vi "BFM.vi"(0 "in 0":T2, 1 "in 1":T2, 2 "in 2":T2, 3 "in 3":T2, 4 "in 4":T2, 5 "in 5":T2, 6 "in 6":T2, 7 "in 7":T2, 8 "in 8":T2, 9 "in 9":T2, 10 "in 10":T2, 11 "in 11":T2, 12 "in 12":T2, 13 "in 13":T2, 14 "in 14":T2, 15 "in 15":T2, 16 "in 16":T2, 17 "in 17":T2, 18 "in 18":T2, 19 "in 19":T2, 20 "in 20":T2, 21 "in 21":T2, 22 "in 22":T2, 23 "in 23":T2, 24 "in 24":T2, 25 "Func":T3) -> (27 "out":T1)   [LabVIEW 2013]
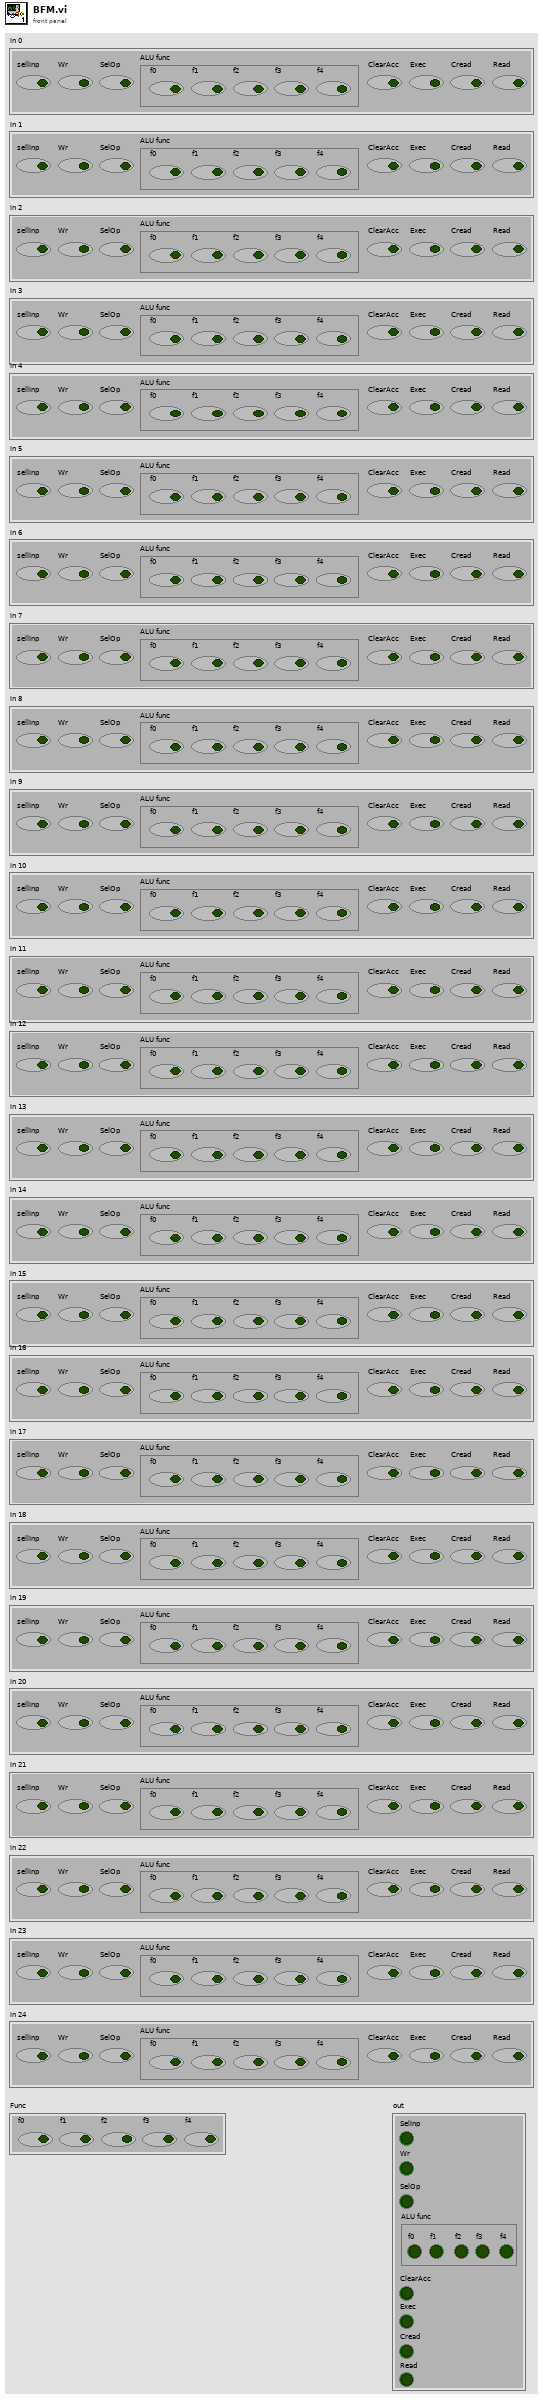
[diagram p1: front panel]
types:
  T1 = cluster{"SelInp":bool, "Wr":bool, "SelOp":bool, "ALU func":cluster{"f0":bool, "f1":bool, "f2":bool, "f3":bool, "f4":bool}, "ClearAcc":bool, "Exec":bool, "Cread":bool, "Read":bool}
  T2 = cluster{"sellInp":bool, "Wr":bool, "SelOp":bool, "ALU func":cluster{"f0":bool, "f1":bool, "f2":bool, "f3":bool, "f4":bool}, "ClearAcc":bool, "Exec":bool, "Cread":bool, "Read":bool}
  T3 = cluster{"f0":bool, "f1":bool, "f2":bool, "f3":bool, "f4":bool}
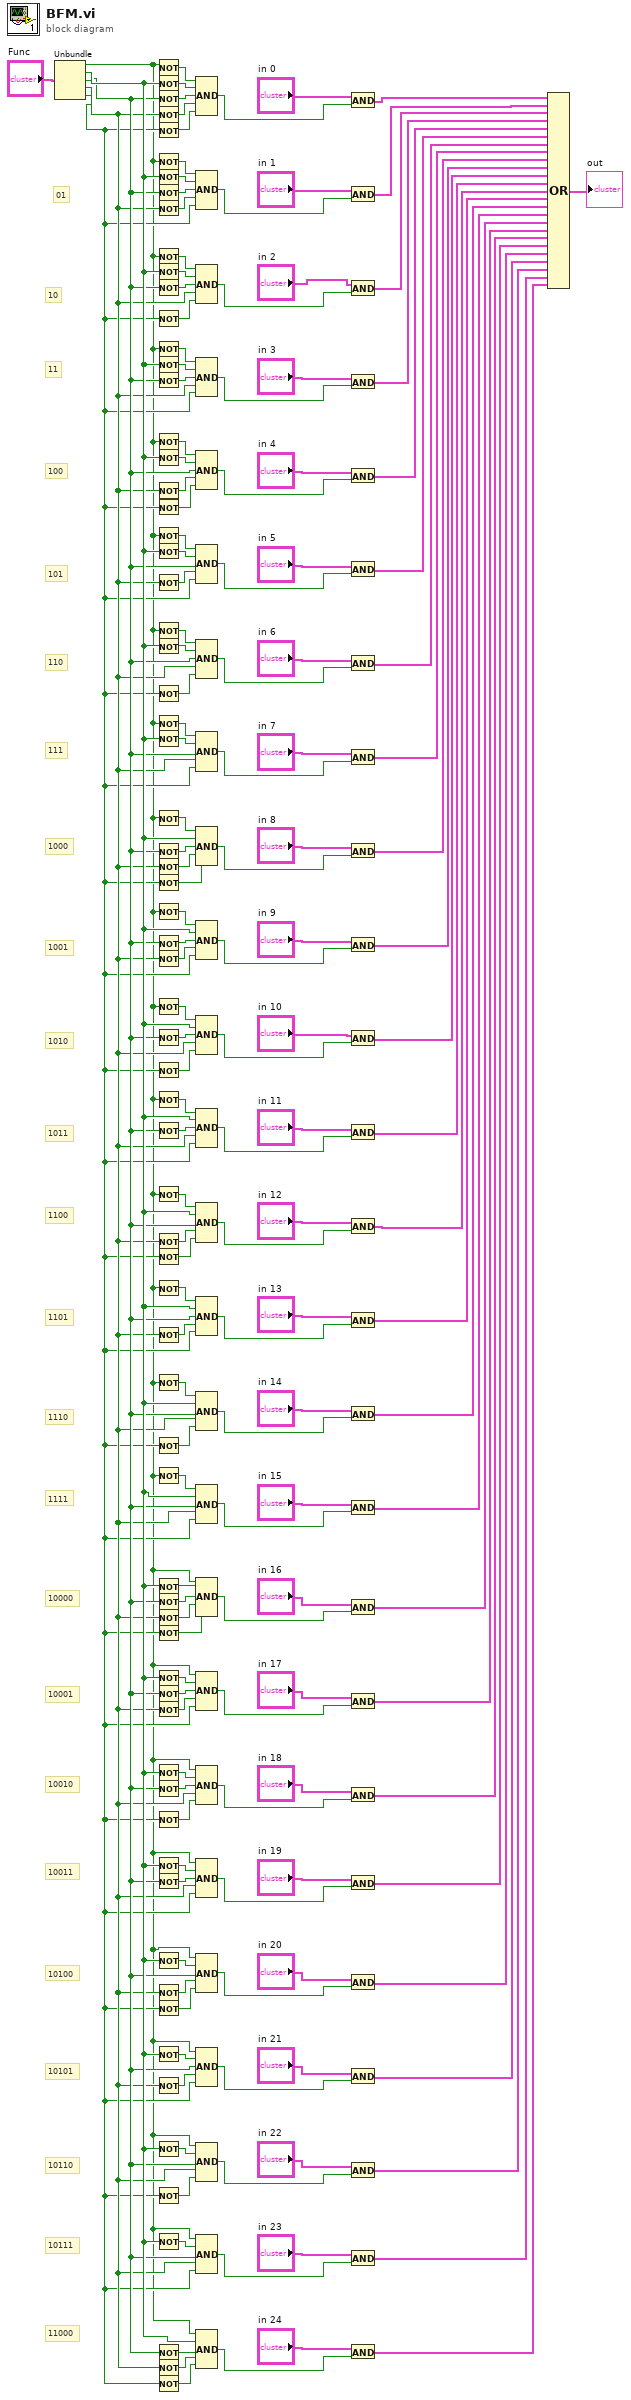
[diagram p0: block diagram]
diagram:
  # "01"
  # "11000"
  # "10111"
  # "10110"
  # "10101"
  # "10100"
  # "10011"
  # "10010"
  # "10001"
  # "10000"
  # "1111"
  # "1110"
  # "1101"
  # "1100"
  # "1011"
  # "1010"
  # "1001"
  # "1000"
  # "111"
  # "110"
  # "101"
  # "100"
  # "11"
  # "10"
  n1 = Unbundle("Func") -> ("f0"=w1:bool, "f1"=w8:bool, "f2"=w4:bool, "f3"=w3:bool, "f4"=w2:bool)
  n2 = Not(x=w1) -> (.not. x?=w94:bool)
  n3 = Not(x=w8) -> (.not. x?=w93:bool)
  n4 = Not(x=w4) -> (.not. x?=w90:bool)
  n5 = Not(x=w3) -> (.not. x?=w91:bool)
  n6 = Not(x=w2) -> (.not. x?=w92:bool)
  n7 = Not(x=w1) -> (.not. x?=w89:bool)
  n8 = Not(x=w8) -> (.not. x?=w88:bool)
  n9 = Not(x=w4) -> (.not. x?=w86:bool)
  n10 = Not(x=w3) -> (.not. x?=w87:bool)
  n11 = Not(x=w1) -> (.not. x?=w85:bool)
  n12 = Not(x=w8) -> (.not. x?=w84:bool)
  n13 = Not(x=w4) -> (.not. x?=w82:bool)
  n14 = Not(x=w2) -> (.not. x?=w83:bool)
  n15 = Not(x=w1) -> (.not. x?=w81:bool)
  n16 = Not(x=w8) -> (.not. x?=w80:bool)
  n17 = Not(x=w4) -> (.not. x?=w79:bool)
  n18 = Not(x=w1) -> (.not. x?=w111:bool)
  n19 = Not(x=w8) -> (.not. x?=w110:bool)
  n20 = Not(x=w3) -> (.not. x?=w26:bool)
  n21 = Not(x=w2) -> (.not. x?=w25:bool)
  n22 = Not(x=w1) -> (.not. x?=w109:bool)
  n23 = Not(x=w8) -> (.not. x?=w108:bool)
  n24 = Not(x=w3) -> (.not. x?=w107:bool)
  n25 = Not(x=w1) -> (.not. x?=w106:bool)
  n26 = Not(x=w8) -> (.not. x?=w105:bool)
  n27 = Not(x=w2) -> (.not. x?=w24:bool)
  n28 = Not(x=w1) -> (.not. x?=w104:bool)
  n29 = Not(x=w8) -> (.not. x?=w103:bool)
  n30 = Not(x=w1) -> (.not. x?=w102:bool)
  n31 = Not(x=w4) -> (.not. x?=w23:bool)
  n32 = Not(x=w3) -> (.not. x?=w22:bool)
  n33 = Not(x=w2) -> (.not. x?=w21:bool)
  n34 = Not(x=w1) -> (.not. x?=w101:bool)
  n35 = Not(x=w4) -> (.not. x?=w99:bool)
  n36 = Not(x=w3) -> (.not. x?=w100:bool)
  n37 = Not(x=w1) -> (.not. x?=w98:bool)
  n38 = Not(x=w4) -> (.not. x?=w97:bool)
  n39 = Not(x=w2) -> (.not. x?=w20:bool)
  n40 = Not(x=w1) -> (.not. x?=w96:bool)
  n41 = Not(x=w4) -> (.not. x?=w95:bool)
  n42 = Not(x=w1) -> (.not. x?=w116:bool)
  n43 = Not(x=w3) -> (.not. x?=w19:bool)
  n44 = Not(x=w2) -> (.not. x?=w18:bool)
  n45 = Not(x=w1) -> (.not. x?=w115:bool)
  n46 = Not(x=w3) -> (.not. x?=w114:bool)
  n47 = Not(x=w1) -> (.not. x?=w113:bool)
  n48 = Not(x=w2) -> (.not. x?=w17:bool)
  n49 = Not(x=w1) -> (.not. x?=w112:bool)
  n50 = Not(x=w8) -> (.not. x?=w16:bool)
  n51 = Not(x=w4) -> (.not. x?=w15:bool)
  n52 = Not(x=w3) -> (.not. x?=w14:bool)
  n53 = Not(x=w2) -> (.not. x?=w13:bool)
  n54 = Not(x=w8) -> (.not. x?=w128:bool)
  n55 = Not(x=w4) -> (.not. x?=w126:bool)
  n56 = Not(x=w3) -> (.not. x?=w127:bool)
  n57 = Not(x=w8) -> (.not. x?=w125:bool)
  n58 = Not(x=w4) -> (.not. x?=w124:bool)
  n59 = Not(x=w2) -> (.not. x?=w12:bool)
  n60 = Not(x=w8) -> (.not. x?=w123:bool)
  n61 = Not(x=w4) -> (.not. x?=w122:bool)
  n62 = Not(x=w8) -> (.not. x?=w121:bool)
  n63 = Not(x=w3) -> (.not. x?=w11:bool)
  n64 = Not(x=w2) -> (.not. x?=w10:bool)
  n65 = Not(x=w8) -> (.not. x?=w120:bool)
  n66 = Not(x=w3) -> (.not. x?=w119:bool)
  n67 = Not(x=w8) -> (.not. x?=w118:bool)
  n68 = Not(x=w2) -> (.not. x?=w9:bool)
  n69 = Not(x=w8) -> (.not. x?=w117:bool)
  n70 = Not(x=w4) -> (.not. x?=w7:bool)
  n71 = Not(x=w3) -> (.not. x?=w6:bool)
  n72 = Not(x=w2) -> (.not. x?=w5:bool)
  n73 = Compound Arithmetic op=AND(w94, w93, w90, w91, w92) -> (w53:bool)
  n74 = Compound Arithmetic op=AND(w89, w88, w86, w87, w2) -> (w54:bool)
  n75 = Compound Arithmetic op=AND(w85, w84, w82, w3, w83) -> (w55:bool)
  n76 = Compound Arithmetic op=AND(w81, w80, w79, w3, w2) -> (w56:bool)
  n77 = Compound Arithmetic op=AND(w111, w110, w4, w26, w25) -> (w57:bool)
  n78 = Compound Arithmetic op=AND(w109, w108, w4, w107, w2) -> (w58:bool)
  n79 = Compound Arithmetic op=AND(w106, w105, w4, w3, w24) -> (w59:bool)
  n80 = Compound Arithmetic op=AND(w104, w103, w4, w3, w2) -> (w60:bool)
  n81 = Compound Arithmetic op=AND(w102, w8, w23, w22, w21) -> (w61:bool)
  n82 = Compound Arithmetic op=AND(w101, w8, w99, w100, w2) -> (w62:bool)
  n83 = Compound Arithmetic op=AND(w98, w8, w97, w3, w20) -> (w63:bool)
  n84 = Compound Arithmetic op=AND(w96, w8, w95, w3, w2) -> (w64:bool)
  n85 = Compound Arithmetic op=AND(w116, w8, w4, w19, w18) -> (w65:bool)
  n86 = Compound Arithmetic op=AND(w115, w8, w4, w114, w2) -> (w66:bool)
  n87 = Compound Arithmetic op=AND(w113, w8, w4, w3, w17) -> (w67:bool)
  n88 = Compound Arithmetic op=AND(w112, w8, w4, w3, w2) -> (w68:bool)
  n89 = Compound Arithmetic op=AND(w1, w16, w15, w14, w13) -> (w69:bool)
  n90 = Compound Arithmetic op=AND(w1, w128, w126, w127, w2) -> (w70:bool)
  n91 = Compound Arithmetic op=AND(w1, w125, w124, w3, w12) -> (w71:bool)
  n92 = Compound Arithmetic op=AND(w1, w123, w122, w3, w2) -> (w72:bool)
  n93 = Compound Arithmetic op=AND(w1, w121, w4, w11, w10) -> (w73:bool)
  n94 = Compound Arithmetic op=AND(w1, w120, w4, w119, w2) -> (w74:bool)
  n95 = Compound Arithmetic op=AND(w1, w118, w4, w3, w9) -> (w75:bool)
  n96 = Compound Arithmetic op=AND(w1, w117, w4, w3, w2) -> (w76:bool)
  n97 = Compound Arithmetic op=AND(w1, w8, w7, w6, w5) -> (w77:bool)
  n98 = And(x="in 0", y=w53) -> (x .and. y?=w52:T2)
  n99 = And(x="in 1", y=w54) -> (x .and. y?=w51:T2)
  n100 = And(x="in 2", y=w55) -> (x .and. y?=w50:T2)
  n101 = And(x="in 3", y=w56) -> (x .and. y?=w49:T2)
  n102 = And(x="in 4", y=w57) -> (x .and. y?=w48:T2)
  n103 = And(x="in 5", y=w58) -> (x .and. y?=w47:T2)
  n104 = And(x="in 6", y=w59) -> (x .and. y?=w46:T2)
  n105 = And(x="in 7", y=w60) -> (x .and. y?=w45:T2)
  n106 = And(x="in 8", y=w61) -> (x .and. y?=w44:T2)
  n107 = And(x="in 9", y=w62) -> (x .and. y?=w43:T2)
  n108 = And(x="in 10", y=w63) -> (x .and. y?=w42:T2)
  n109 = And(x="in 11", y=w64) -> (x .and. y?=w41:T2)
  n110 = And(x="in 12", y=w65) -> (x .and. y?=w40:T2)
  n111 = And(x="in 13", y=w66) -> (x .and. y?=w39:T2)
  n112 = And(x="in 14", y=w67) -> (x .and. y?=w38:T2)
  n113 = And(x="in 15", y=w68) -> (x .and. y?=w37:T2)
  n114 = And(x="in 16", y=w69) -> (x .and. y?=w36:T2)
  n115 = And(x="in 17", y=w70) -> (x .and. y?=w35:T2)
  n116 = And(x="in 18", y=w71) -> (x .and. y?=w34:T2)
  n117 = And(x="in 19", y=w72) -> (x .and. y?=w33:T2)
  n118 = And(x="in 20", y=w73) -> (x .and. y?=w32:T2)
  n119 = And(x="in 21", y=w74) -> (x .and. y?=w31:T2)
  n120 = And(x="in 22", y=w75) -> (x .and. y?=w30:T2)
  n121 = And(x="in 23", y=w76) -> (x .and. y?=w29:T2)
  n122 = And(x="in 24", y=w77) -> (x .and. y?=w28:T2)
  n123 = Compound Arithmetic op=OR(w52, w51, w50, w49, w48, w47, w46, w45, w44, w43, w42, w41, w40, w39, w38, w37, w36, w35, w34, w33, w32, w31, w30, w29, w28) -> (→"out":T2)
